vi "OAT Even Time or Speed Segment.vi"   [LabVIEW 2017, in "SoundVib_OAUtility.lvlib"]
doc: "Divides an input signal into even-time segments or even-speed intervals. The input signal of this VI can be an even-angle signal or an XY signal. When you use this VI to divide an XY signal, the XY signal can be only the output of the OAT Order Magnitude and Phase VI or OAT Overall Level Plot VI. Wire data to the <B>even-angle signal</B> input to determine the polymorphic instance to use or manually select the instance."
uses:
  <vilib>/addons/Sound and Vibration/Order Analysis/Utility/SoundVib_OAUtility.lvlib
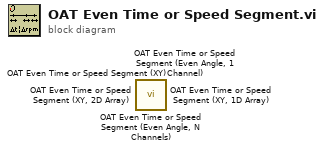
[diagram p0: block diagram]
diagram:
  n1 = call <vilib>:"OAT Even Time or Speed Segment (Even Angle, N Channels).vi"() -> ()  [unwired: 10 in, 6 out]
  n2 = call <vilib>:"OAT Even Time or Speed Segment (Even Angle, 1 Channel).vi"() -> ()  [unwired: 10 in, 6 out]
  n3 = call <vilib>:"OAT Even Time or Speed Segment (XY, 2D Array).vi"() -> ()  [unwired: 11 in, 5 out]
  n4 = call <vilib>:"OAT Even Time or Speed Segment (XY, 1D Array).vi"() -> ()  [unwired: 11 in, 5 out]
  n5 = call <vilib>:"OAT Even Time or Speed Segment (XY).vi"() -> ()  [unwired: 11 in, 5 out]
